vi "Create 3D Axes.vi"(1 "Cluster":T1) -> ()   [LabVIEW 2010]
uses:
  <vilib>/picture/3D Picture Control/NI_3D Picture Control.lvlib
panel:
  out "Z 2":refnum<vi>
  out "Y 2":refnum<vi>
  out "X 2":refnum<vi>
  out "Trans 3":refnum<vi>
  out "Trans 2":refnum<vi>
  out "Transformation Object":refnum<vi>
  out "X":refnum<vi>
  out "Y":refnum<vi>
  out "Z":refnum<vi>
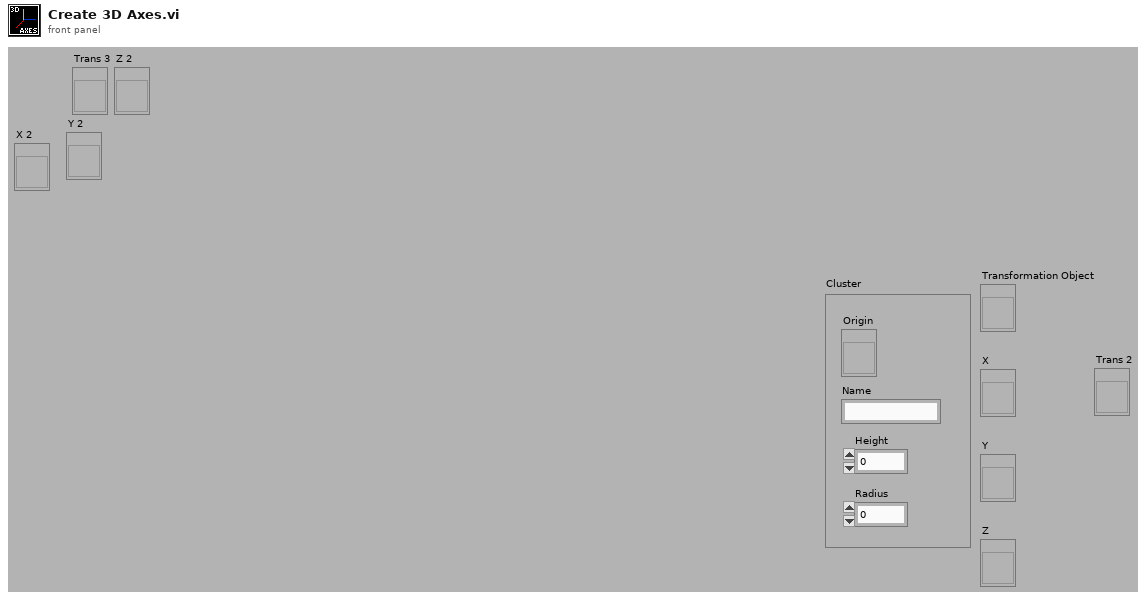
[diagram p1: front panel]
types:
  T1 = cluster{"Origin":refnum<vi>, "Name":string, "Height":sgl, "Radius":sgl}
  T2 = cluster{"Red":sgl, "Green":sgl, "Blue":sgl, "Alpha":sgl}
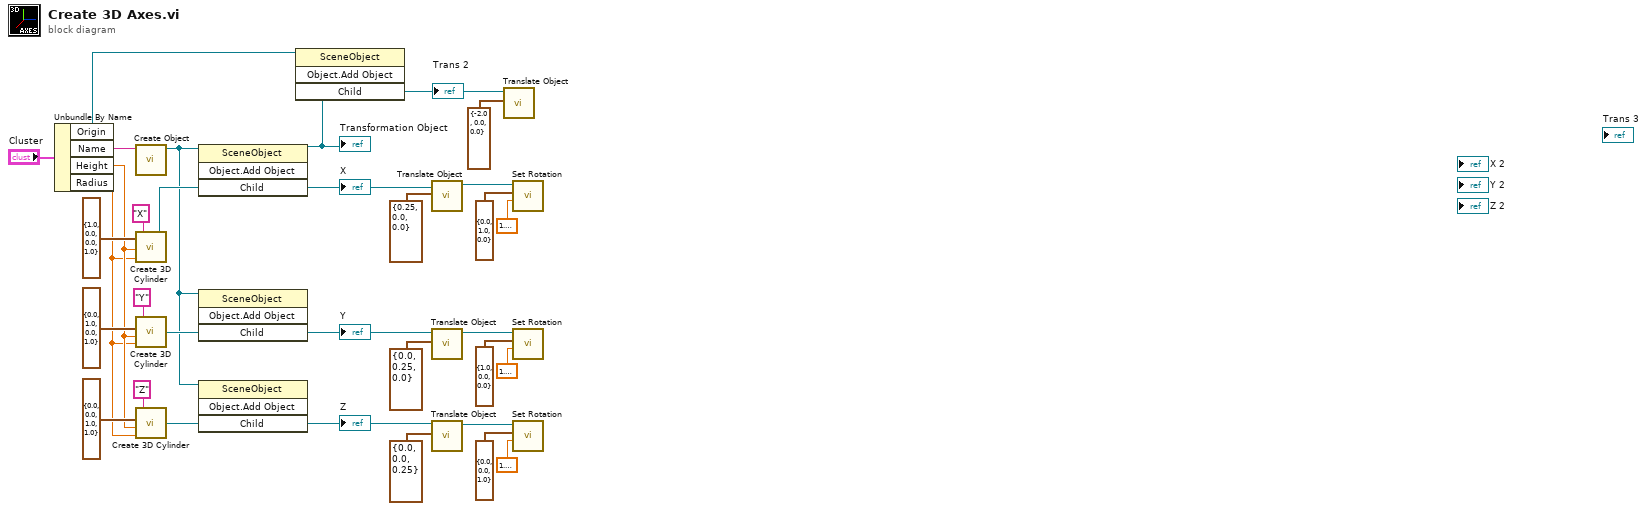
[diagram p0: block diagram]
diagram:
  n1 = Unbundle By Name("Cluster") -> ("Origin"=w19:refnum<vi>, "Name"=w22:string, "Height"=w21:sgl, "Radius"=w20:sgl)
  n2 = call <vilib>:"Create Object.vi"("Name"=w22) -> ("Scene:New Object"=w24:refnum<vi>)  [unwired: 9 in, 1 out]
  n3 = call "Create 3D Cylinder.vi"("Radius"=w20, "Height"=w21, "Color"=T2 {"Red"=1.0, "Green"=0.0, "Blue"=0.0, "Alpha"=1.0}, "Name"="X") -> ("Scene:New Object"=w26:refnum<vi>)
  n4 = call "Create 3D Cylinder.vi"("Radius"=w20, "Height"=w21, "Color"=T2 {"Red"=0.0, "Green"=1.0, "Blue"=0.0, "Alpha"=1.0}, "Name"="Y") -> ("Scene:New Object"=w29:refnum<vi>)
  n5 = call "Create 3D Cylinder.vi"("Radius"=w20, "Height"=w21, "Color"=T2 {"Red"=0.0, "Green"=0.0, "Blue"=1.0, "Alpha"=1.0}, "Name"="Z") -> ("Scene:New Object"=w32:refnum<vi>)
  n6 = invoke class="SceneObject" method="Object.Add Object"(reference=w24, "Child"=w26) -> (reference out=w18:refnum<vi>, "Child"=w3:refnum<vi>)  [unwired: 2 in, 2 out]
  "X" <- w3
  "Transformation Object" <- w18
  n7 = invoke class="SceneObject" method="Object.Add Object"(reference=w24, "Child"=w29) -> ("Child"=w2:refnum<vi>)  [unwired: 2 in, 3 out]
  "Y" <- w2
  n8 = invoke class="SceneObject" method="Object.Add Object"(reference=w24, "Child"=w32) -> ("Child"=w1:refnum<vi>)  [unwired: 2 in, 3 out]
  "Z" <- w1
  n9 = invoke class="SceneObject" method="Object.Add Object"(reference=w19, "Child"=w18) -> ("Child"=w4:refnum<vi>)  [unwired: 2 in, 3 out]
  "Trans 2" <- w4
  n10 = call <vilib>:"Translate Object.vi"("Translation"=cluster{"X":sgl, "Y":sgl, "Z":sgl} {"X"=0.25, "Y"=0.0, "Z"=0.0} ("Axis"), "Scene.Object In"=w3) -> ("Scene.Object Out"=w14:refnum<vi>)  [unwired: 8 in, 1 out]
  n11 = call <vilib>:"Translate Object.vi"("Translation"=cluster{"X":sgl, "Y":sgl, "Z":sgl} {"X"=0.0, "Y"=0.25, "Z"=0.0} ("Axis"), "Scene.Object In"=w2) -> ("Scene.Object Out"=w15:refnum<vi>)  [unwired: 8 in, 1 out]
  n12 = call <vilib>:"Translate Object.vi"("Translation"=cluster{"X":sgl, "Y":sgl, "Z":sgl} {"X"=0.0, "Y"=0.0, "Z"=0.25} ("Axis"), "Scene.Object In"=w1) -> ("Scene.Object Out"=w16:refnum<vi>)  [unwired: 8 in, 1 out]
  n13 = call <vilib>:"Translate Object.vi"("Translation"=cluster{"X":sgl, "Y":sgl, "Z":sgl} {"X"=-2.0, "Y"=0.0, "Z"=0.0} ("Axis"), "Scene.Object In"=w4) -> ()  [unwired: 8 in, 2 out]
  n14 = call <vilib>:"Set Rotation.vi"("Angle"=1.5707963267948966, "Axis"=cluster{"X":sgl, "Y":sgl, "Z":sgl} {"X"=0.0, "Y"=1.0, "Z"=0.0} ("Axis 2"), "Scene Object"=w14) -> ()  [unwired: 7 in, 2 out]
  n15 = call <vilib>:"Set Rotation.vi"("Angle"=1.5707963267948966, "Axis"=cluster{"X":sgl, "Y":sgl, "Z":sgl} {"X"=1.0, "Y"=0.0, "Z"=0.0} ("Axis 2"), "Scene Object"=w15) -> ()  [unwired: 7 in, 2 out]
  n16 = call <vilib>:"Set Rotation.vi"("Angle"=1.5707963267948966, "Axis"=cluster{"X":sgl, "Y":sgl, "Z":sgl} {"X"=0.0, "Y"=0.0, "Z"=1.0} ("Axis 2"), "Scene Object"=w16) -> ()  [unwired: 7 in, 2 out]
